vi "SpaceTimeConversion.vi"(1 "Conversion Type: T : Distance to Time\n                             F : Time to Distance":bool, 2 "Time IN (ps)":dbl[](array[numeric]), 3 "Distance IN (mm)":dbl[](array[numeric]), 4 "Zero Position":dbl) -> (0 "Time OUT (ps) / Distance OUT (mm)":dbl[](array[numeric]))   [LabVIEW 2013]
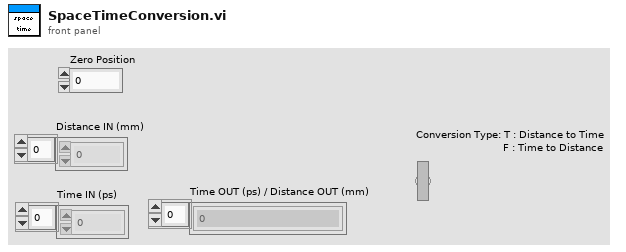
[diagram p1: front panel]
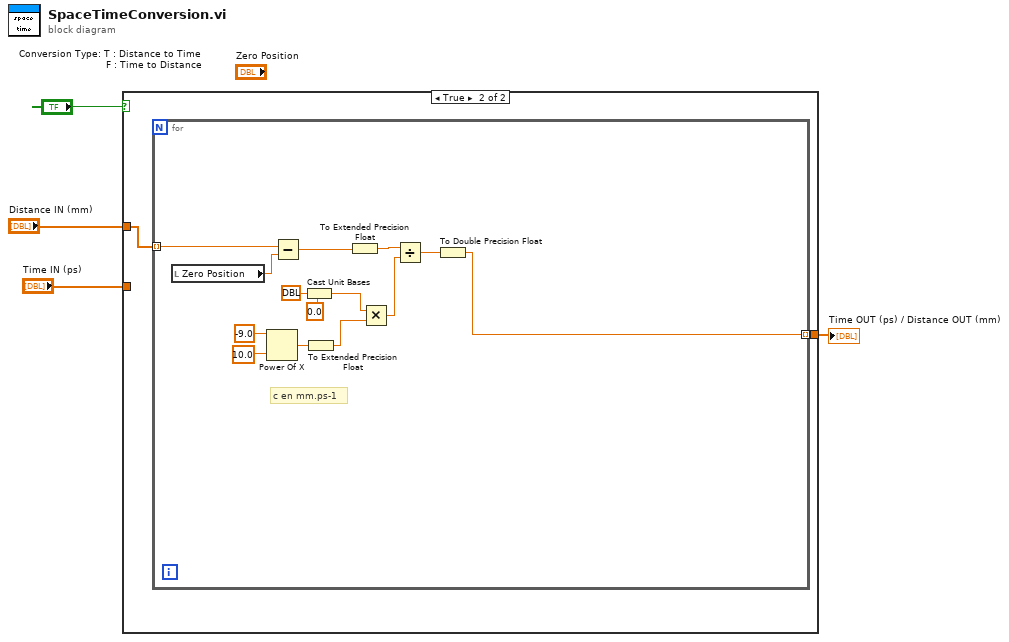
[diagram p0: block diagram]
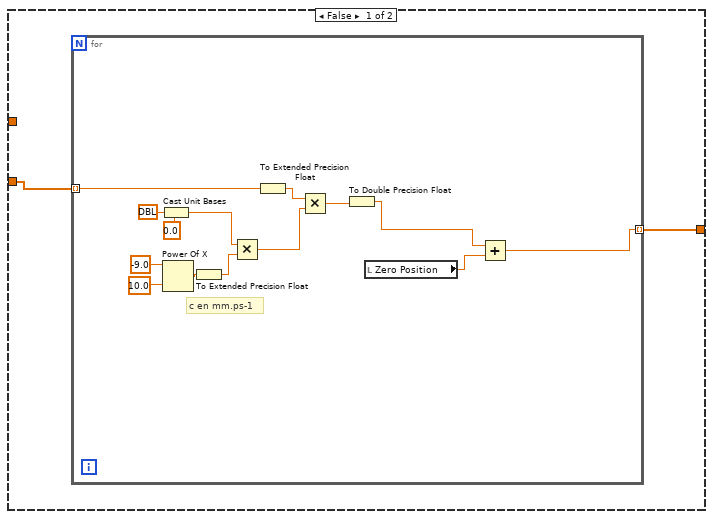
[diagram p2: hidden frame]
diagram:
  n1 = case shown="True" "Conversion Type: T : Distance to Time\n                             F : Time to Distance" {
    tunnel: "Time IN (ps)" -> [w6 _]
    tunnel: "Distance IN (mm)" -> [_ w21]
    tunnel: [w5 w22] -> w2
    frame False {
      n2 = for {
        tunnel: w6 -> [w10] mode=indexing
        tunnel: [w7] -> w5 mode=indexing
        # "c en mm.ps-1"
        n3 = Cast Unit Bases(0:ext[unit] 299792458.0, 1:0.0 ("unité (aucune)")) -> (2:w14:ext)
        n4 = Power Of X(1:10.0 ("x"), 2:-9.0 ("y")) -> (0:w16:dbl)
        n5 = To Extended Precision Float(1:w16) -> (0:w13:ext)
        n6 = Multiply(x=w14, y=w13) -> (x*y=w12:ext)
        n7 = To Extended Precision Float(1:w10) -> (0:w15:ext)
        n8 = Multiply(x=w15, y=w12) -> (x*y=w11:ext)
        n9 = To Double Precision Float(number=w11) -> (double precision float=w8:dbl)
        n10 = local read "Zero Position"() -> (w9:dbl)
        n11 = Add(x=w8, y=w9) -> (x+y=w7:dbl)
      }
    }
    frame True {
      n12 = for {
        tunnel: [w36] -> w22 mode=indexing
        tunnel: w21 -> [w24] mode=indexing
        # "c en mm.ps-1"
        n13 = local read "Zero Position"() -> (w25:dbl)
        n14 = Power Of X(1:10.0 ("x"), 2:-9.0 ("y")) -> (0:w30:dbl)
        n15 = Subtract(x=w24, y=w25) -> (x-y=w23:dbl)
        n16 = Cast Unit Bases(0:ext[unit] 299792458.0, 1:0.0 ("unité (aucune)")) -> (2:w29:ext)
        n17 = To Extended Precision Float(1:w30) -> (0:w28:ext)
        n18 = To Extended Precision Float(1:w23) -> (0:w31:ext)
        n19 = Multiply(x=w29, y=w28) -> (x*y=w27:ext)
        n20 = Divide(x=w31, y=w27) -> (x/y=w26:ext)
        n21 = To Double Precision Float(number=w26) -> (double precision float=w36:dbl)
      }
    }
  }
  "Time OUT (ps) / Distance OUT (mm)" <- w2
